vi "Create Default Attributes.vi"(5 "Unique ID":string, 7 "Process Executive Ref":refnum<data-value>, 11 "Start Pre-Soak in":refnum<class "Start Pre-Soak.lvclass">) -> (3 "Start Pre-Soak out":refnum<class "Start Pre-Soak.lvclass">)   [LabVIEW 2019, in "Start Pre-Soak.lvclass"]
uses:
  <vilib>/gpm_packages/@cs/Car-wash/Source/Process Steps/Start Pre-Soak/Start Pre-Soak.lvclass
  <vilib>/gpm_packages/@cs/test-executive/Source/Test Executive/ITestExecutive/ITest Executive.lvclass
  f4bb12f1-1f96-43b7-9c53-8c7d6c59b68a.vi
  <vilib>/Utility/error.llb/Error Cluster From Error Code.vi
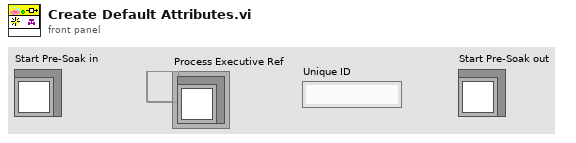
[diagram p1: front panel]
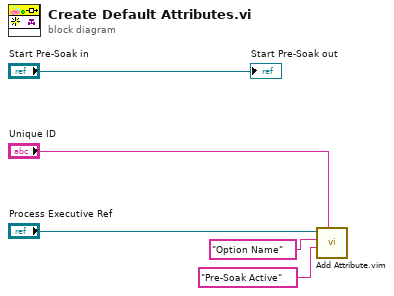
[diagram p0: block diagram]
diagram:
  n1 = call "Add Attribute.vim"("ID"="Unique ID", "Attribute"="Pre-Soak Active" ("Item Name"), "Attribute Name"="Option Name" ("Item Name"), "Test Executive Ref"="Process Executive Ref") -> ()  [unwired: 4 in, 4 out]
  "Start Pre-Soak out" <- "Start Pre-Soak in"
